vi "Temperature Logger.vi"() -> ()   [LabVIEW 2018]
uses:
  <vilib>/Analysis/baseanly.llb/Mean (DBL).vi
  <vilib>/Analysis/NI_AALBase.lvlib
panel:
  out "Mean Temp":dbl
  out "Min Temp":dbl
  out "Max Temp":dbl
  in  "stop":bool
  out "Current Data":dbl(slide) scale=0.0..100.0
  out "Current Index":dbl
  in  "Temp Scale":bool
  # "Deg C"
  # "Deg F"
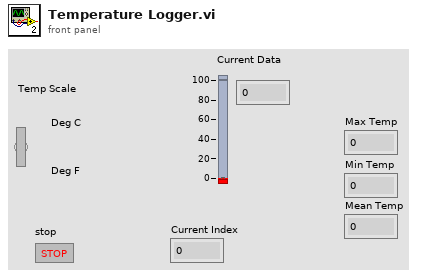
[diagram p1: front panel]
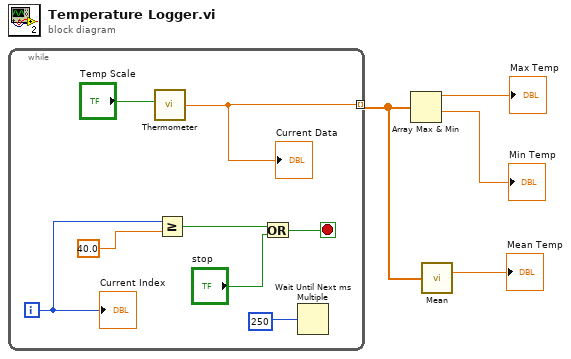
[diagram p0: block diagram]
diagram:
  n1 = while {
    tunnel: [w11] -> w2 mode=indexing
    i -> [w9]
    stop <- w6 stop-if-true
    n2 = call "Thermometer.vi"("Temp Scale"="Temp Scale") -> ("Temperature"=w11:dbl)
    "Current Data" <- w11
    n3 = Greater Or Equal?(x=w9, y=40.0) -> (x >= y?=w7:bool)
    n4 = Or(x=w7, y="stop") -> (x .or. y?=w6:bool)
    n5 = Wait Until Next ms Multiple(millisecond multiple=250) -> ()  [unwired: 1 out]
    "Current Index" <- w9
  }
  n6 = Array Max & Min(array=w2) -> (max value=→"Max Temp":dbl, min value=→"Min Temp":dbl)  [unwired: 2 out]
  n7 = call-poly <vilib>:"Mean.vi"("X"=w2) -> ("mean"=→"Mean Temp":dbl)  [unwired: 1 out]
